vi "plot_pixel_cross_section.vi"(8 "error in (no error)":errorcluster, 10 "avg-data-row":dbl[](array[numeric]), 11 "XYGraph":refnum<vi>) -> (0 "error out":errorcluster, 3 "figure (out)":refnum<vi>)   [LabVIEW 2017]
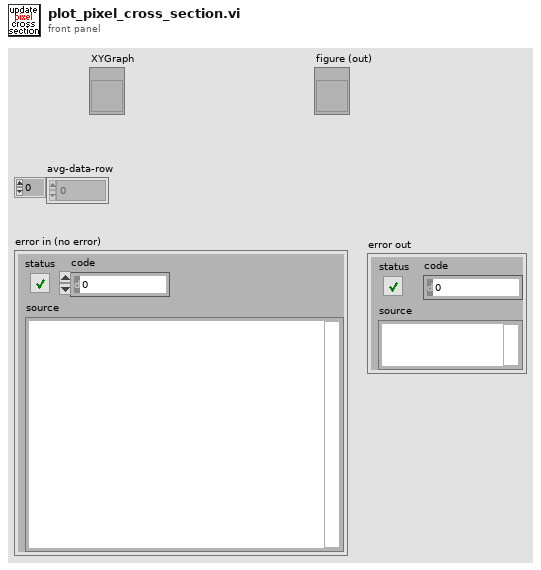
[diagram p1: front panel]
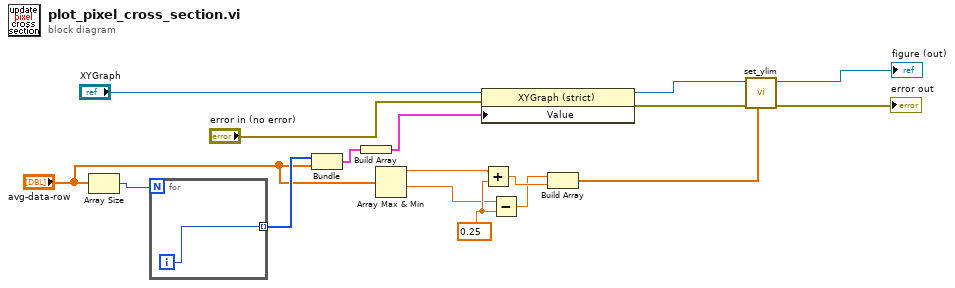
[diagram p0: block diagram]
diagram:
  w14 = 0.25
  n1 = Array Size(array="avg-data-row") -> (size(s)=w7:i32)
  n2 = for {
    N: w7 -> [_]
    tunnel: [w18] -> w6 mode=indexing
    i -> [w18]
  }
  n3 = Bundle(w6, "avg-data-row"="avg-data-row") -> (w5:cluster{i32[], "avg-data-row":dbl[]})  [unwired: 1 in]
  n4 = Build Array(w5) -> (w4:cluster{i32[], "avg-data-row":dbl[]}[])
  n5 = Array Max & Min(array="avg-data-row") -> (max value=w12:dbl, min value=w13:dbl)  [unwired: 2 out]
  n6 = property on="Property Node" class="XYGraph (strict)"(reference="XYGraph", error in="error in (no error)", "Value"=w4) -> (reference out=w16:refnum<vi>, error out=w17:errorcluster)
  n7 = Add(x=w12, y=w14) -> (x+y=w2:dbl)
  n8 = Subtract(x=w13, y=w14) -> (x-y=w1:dbl)
  n9 = Build Array(w1, w2) -> (w15:dbl[])
  n10 = call "set_ylim.vi"("ylim"=w15, "error in"=w17, "figure (in)"=w16) -> ("error out"=→"error out":errorcluster, "figure (out)"=→"figure (out)":refnum<vi>)  [unwired: 7 in]
